vi "SetVelocity(rps).vi"(7 "Units":enum16{"r/s", "r/m"}(ring), 8 "error in (no error)":errorcluster, 10 "velocity":dbl, 11 "Motor Base in":refnum<class "Motor Base.lvclass">) -> (0 "error out":errorcluster, 3 "Motor Base out":refnum<class "Motor Base.lvclass">)   [LabVIEW 2016, in "Motor Base.lvlib" / "Motor Base.lvclass"]
uses:
  Motor Base.lvclass
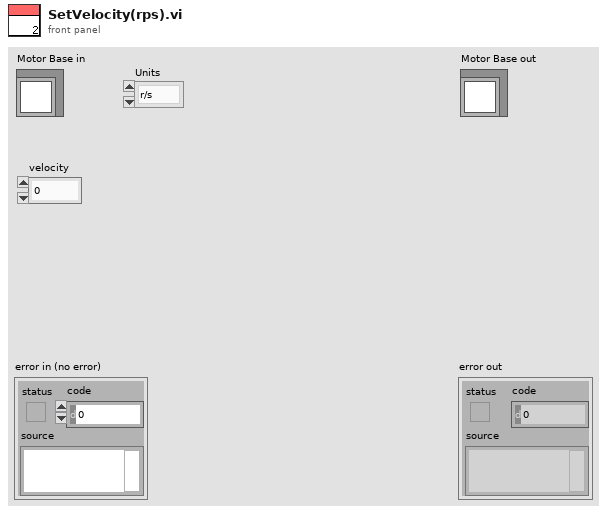
[diagram p1: front panel]
types:
  T1 = cluster{"Modes of operation":i8, "Feed(pulse)":u32, "Max motor speed(r/min)":u32, "Max torque(0.1%)":u16, "Min position limit(pulse)":i32, "Max position limit(pulse)":i32}
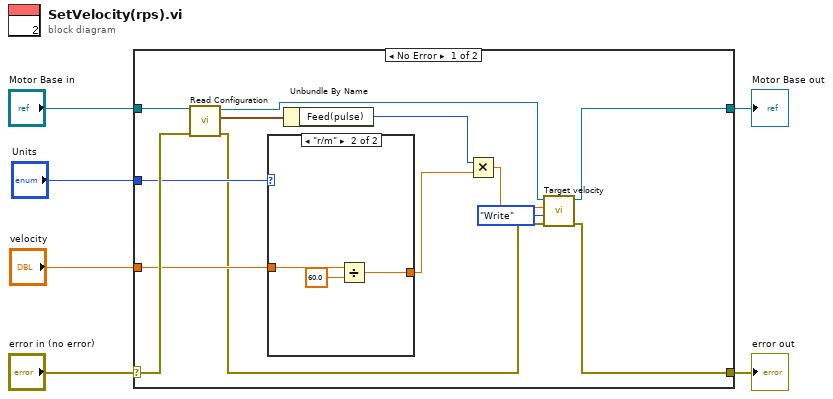
[diagram p0: block diagram]
diagram:
  n1 = case shown="No Error" "error in (no error)" {
    selector: "error in (no error)" -> [w18 w25]
    tunnel: [w9 w25] -> w5
    tunnel: [w8 w24] -> w3
    tunnel: "Motor Base in" -> [w19 w24]
    tunnel: "Units" -> [w16 _]
    tunnel: "velocity" -> [w15 _]
    frame No Error {
      n2 = call-dynamic "Read Configuration.vi"("error in (no error)"=w18, "Motor Base in"=w19) -> ("error out"=w10:errorcluster, "Configuration"=w17:T1, "Motor Base out"=w12:refnum<class "Motor Base.lvclass">)  [unwired: 7 in]
      n3 = case shown="\"r/m\"" w16 {
        tunnel: w15 -> [w20 w23]
        tunnel: [w20 w21] -> w13
        frame "r/s", Default {
        }
        frame "r/m" {
          n4 = Divide(x=w23, y=60.0) -> (x/y=w21:dbl)
        }
      }
      n5 = Unbundle By Name(w17) -> ("Feed(pulse)"=w14:u32)
      n6 = Multiply(x=w14, y=w13) -> (x*y=w11:dbl)
      n7 = call-dynamic "Target velocity.vi"("error in"=w10, "W/R"=enum16{"Write", "Read"}."Write", "Data"=w11, "Motor Base in"=w12) -> ("error out"=w9:errorcluster, "Motor Base out"=w8:refnum<class "Motor Base.lvclass">)  [unwired: 5 in, 1 out]
    }
    frame Error {
    }
  }
  "error out" <- w5
  "Motor Base out" <- w3
